vi "RSZVB Set Pulse Generator Master Channel.vi"(8 "error in (no error)":errorcluster {"code" format="%.0x"}, 9 "Master Channel (1)":i32=1, 11 "VISA resource name":refnum<visa-resource-name>) -> (0 "error out":errorcluster {"code" format="%.0x"}, 3 "VISA resource name out":refnum<visa-resource-name>)   [LabVIEW 2011]
doc: "This VI selects the master channel for CONTinuous pulse mode (rszvb_SetPulseGeneratorMode).\n\nNote(s):\n\n(1) This VI is available only with option R&S ZVA-K27.\n\nRemote-control command(s):\n[SENSe<Ch>:]PULSe:GENerator<gen_no>:MCHannel"
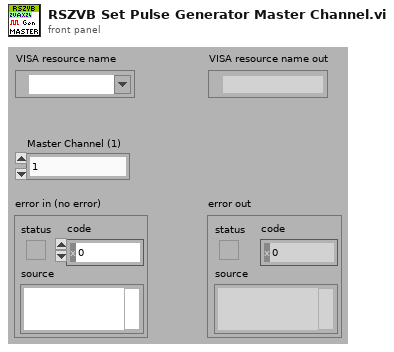
[diagram p1: front panel]
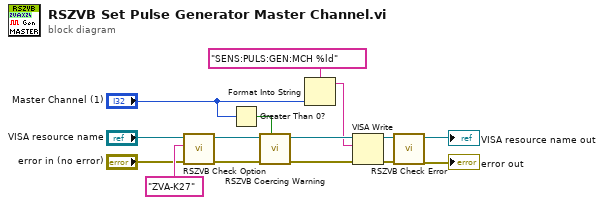
[diagram p0: block diagram]
diagram:
  n1 = call "RSZVB Check Option.vi"("error in (no error)"="error in (no error)", "Options"="ZVA-K27", "VISA session"="VISA resource name") -> ("error out"=w1:errorcluster, "dup VISA session"=w3:refnum<visa-resource-name>)  [unwired: 7 in]
  n2 = Greater Than 0?(x="Master Channel (1)") -> (x > 0?=w9:bool)
  n3 = call "RSZVB Coercing Warning.vi"("In Range?"=w9, "error in (no error)"=w1, "VISA session"=w3) -> ("error out"=w13:errorcluster, "dup VISA session"=w14:refnum<visa-resource-name>)  [unwired: 7 in]
  n4 = Format Into String(format string="SENS:PULS:GEN:MCH %ld", "Master Channel (1)") -> (resulting string=w10:string)  [unwired: 2 in, 1 out]
  n5 = VISA Write(VISA resource name=w14, write buffer=w10, error in (no error)=w13) -> (VISA resource name out=w11:refnum<visa-resource-name>, error out=w12:errorcluster)  [unwired: 1 out]
  n6 = call "RSZVB Check Error.vi"("error in (no error)"=w12, "VISA session"=w11) -> ("error out"=→"error out":errorcluster, "dup VISA session"=→"VISA resource name out":refnum<visa-resource-name>)  [unwired: 8 in]
